vi "direct host fetch.vi"() -> ()   [LabVIEW 2013]
uses:
  <instrlib>/niScope/Controls/niScope vertical coupling.ctl
  <instrlib>/niScope/Configure/Trigger/niScope Configure Trigger Immediate.vi
  <instrlib>/niScope/Acquire/Fetch/niScope Fetch Binary 16.vi
panel:
  out "error out":errorcluster
  out "Waveform Graph":i16[](graph)
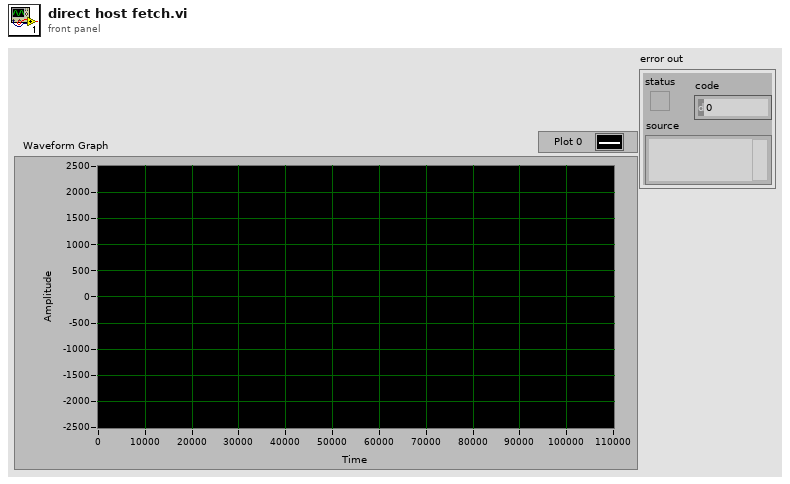
[diagram p1: front panel]
types:
  T1 = typedef "niScope vertical coupling.ctl" = i32
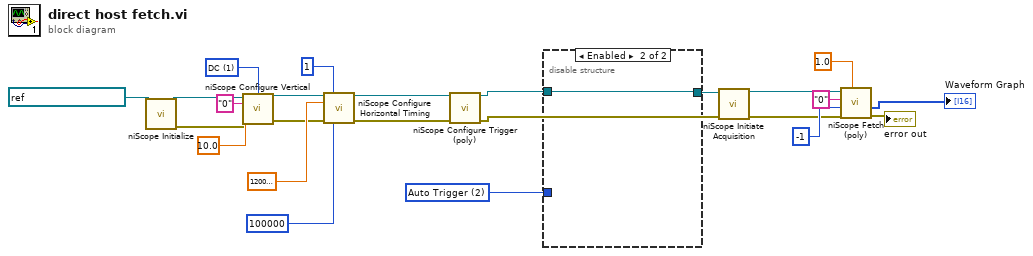
[diagram p0: block diagram]
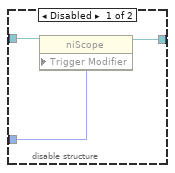
[diagram p2: hidden frame]
diagram:
  w1 = 2 items=["None"=1, "Auto Trigger"=2] ("Triggering:Trigger Modifier")
  w21 = T1 1 items=["AC", "DC", "Ground"] ("vertical coupling")
  n1 = call <instrlib>:"niScope Initialize.vi"("resource name"=refnum<k15> "Dev1") -> ("instrument handle"=w23:refnum<k15>, "error out"=w9:errorcluster)  [unwired: 13 in]
  n2 = call <instrlib>:"niScope Configure Vertical.vi"("instrument handle"=w23, "vertical coupling"=w21, "channels"="0", "vertical range"=10.0, "error in"=w9) -> ("instrument handle out"=w20:refnum<k15>, "error out"=w8:errorcluster)  [unwired: 9 in]
  n3 = call <instrlib>:"niScope Configure Horizontal Timing.vi"("instrument handle"=w20, "number of records"=1, "min sample rate"=1200000000.0, "error in"=w8, "min record length"=100000) -> ("instrument handle out"=w18:refnum<k15>, "error out"=w7:errorcluster)  [unwired: 9 in]
  n4 = call-poly <instrlib>:"niScope Configure Trigger (poly).vi"("instrument handle"=w18, "error in"=w7) -> ("instrument handle out"=w3:refnum<k15>, "error out"=w6:errorcluster)  [unwired: 12 in]
  n5 = disable-structure shown="Enabled" {
    disable-tunnel: w3 -> [w27 w28]
    disable-tunnel: [w26 w28] -> w2
    disable-tunnel: w1 -> [w25 _]
    frame Disabled {
      n6 = property class="niScope"(reference=w27, "Trigger Modifier"=w25) -> (reference out=w26:refnum<k15>)  [unwired: 1 in, 1 out]
    }
    frame Enabled {
    }
  }
  n7 = call <instrlib>:"niScope Initiate Acquisition.vi"("instrument handle"=w2, "error in"=w6) -> ("instrument handle out"=w17:refnum<k15>, "error out"=w5:errorcluster)  [unwired: 12 in]
  n8 = call-poly <instrlib>:"niScope Fetch (poly).vi"("timeout"=1.0, "error in"=w5, "numSamples"=-1, "channels"="0", "instrument handle"=w17) -> ("error out"=→"error out":errorcluster, "wfm"=→"Waveform Graph":i16[])  [unwired: 3 in, 2 out]
